vi "event_to_dom_load_interface.vi"(8 "error in (no error)":errorcluster, 11 "interface":T1) -> (0 "error out":errorcluster)   [LabVIEW 2015, in "lv-interface-dom-nre.lvlib"]
uses:
  lv-interface-dom-nre.lvlib
  lv-interface-sub-common/_controls/interface_selection.ctl
  _controls/event_to_dom_command.ctl
  lv-interface-sub-common/lv-interface-sub-common.lvlib
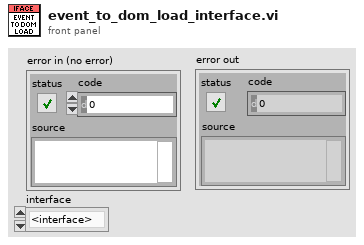
[diagram p1: front panel]
types:
  T1 = typedef "lv-interface-sub-common.lvlib/interface_selection.ctl" = enum16{"<interface>", "sub_interface_1", "sub_interface_2", "<null>"}
  T2 = typedef "lv-interface-dom-nre.lvlib/event_to_dom_command.ctl" = enum16{"<to_dom_cmd>", "load_interface", "die", "<null>"}
  T3 = typedef "lv-interface-dom-nre.lvlib/event_to_dom.ctl" = cluster{"command":T2, "interface":T1, "data":variant}
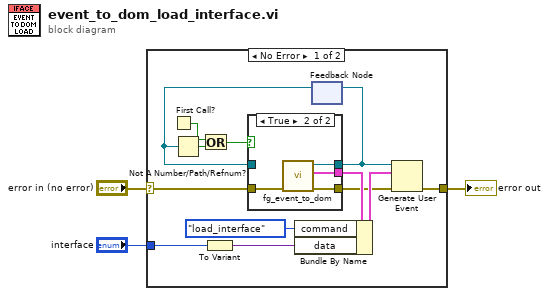
[diagram p0: block diagram]
diagram:
  n1 = case shown="No Error" "error in (no error)" {
    selector: "error in (no error)" -> [w16 w23]
    tunnel: [w11 w23] -> w2
    tunnel: "interface" -> [w5 _]
    frame No Error {
      n2 = First Call?() -> (First Call?: T/F=w7:bool)
      n3 = To Variant(anything=w5) -> (Variant=w4:variant)
      n4 = feedback #1() -> (w9:refnum<user-event>)  [unwired: 1 in]
      n5 = Not A Number/Path/Refnum?(number/path/refnum=w9) -> (NaN/Path/Refnum?=w8:bool)
      n6 = Or(x=w7, y=w8) -> (x .or. y?=w10:bool)
      n7 = case shown="True" w10 {
        tunnel: w16 -> [w17 w22]
        tunnel: [w18 w21] -> w15
        tunnel: [_ w20] -> w14
        tunnel: [w17 w19] -> w12
        tunnel: w9 -> [w18 _]
        frame False {
        }
        frame True {
          n8 = call "fg_event_to_dom.vi"("error in (no error)"=w22) -> ("error out"=w19:errorcluster, "data"=w20:T3, "to_dom"=w21:refnum<user-event>)  [unwired: 8 in]
        }
      }
      n9 = Bundle By Name(cluster=w14, "command"=event_to_dom_command."load_interface", "data"=w4) -> (w13:T3)
      n10 = feedback-in #1(w15) -> ()
      n11 = Generate User Event(user event=w15, event data cluster=w13, error in=w12) -> (error out=w11:errorcluster)  [unwired: 1 in, 1 out]
    }
    frame Error {
    }
  }
  "error out" <- w2
